vi "GetObjectStatus.vi"(0 "reference in":refnum<class "G#RemoteProxy.lvclass">, 2 "simple info (F)":bool, 5 "error in (no error)":errorcluster) -> (8 "full class name":string, 9 "# of users?":i32, 10 "all object names":string[](array[string]), 11 "last user":bool, 12 "# of objects":i32, 13 "class name":string, 14 "reference out":refnum<class "G#RemoteProxy.lvclass">, 15 "not a refnum?":bool, 16 "object name":string, 17 "all refs out":refnum<class "G#Object.lvclass">[](array[class]), 18 "counter?":bool, 19 "error out":errorcluster)   [LabVIEW 2017, in "G#RemoteProxy.lvclass"]
doc: "Returns information about the specified object. If simple info = true, only object info is return and not the arrays of objects.\n\nIf input reference is invalid, only information about the class is returned."
uses:
  G#RemoteProxy.lvclass
  G#Object/G#Object.lvclass
  G#RemoteProxy.lvclass/G#RemoteProxy.ctl
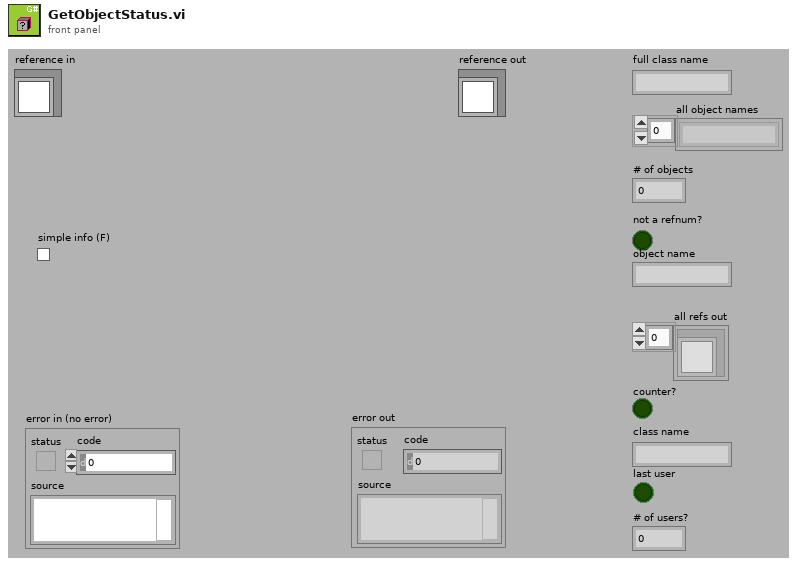
[diagram p1: front panel]
types:
  T1 = typedef "G#RemoteProxy.lvclass/ObjectAttributesRef.ctl" = refnum<data-value>
  T2 = typedef "G#RemoteProxy.lvclass/ObjectAttributesProxy.ctl" = cluster{"class hierarchy":T3[], "class name":string, "lvlib hierarchy":string[], "full class name":string, "id":u32, "owner":string, "RemoteRef":refnum<class "G#Object.lvclass">, "object name":string, "attributes":variant[], "connection ID":refnum<k5>, "address":u32, "occurrence":refnum<k4>, "ProxyClassRef":refnum<class "G#RemoteProxy.lvclass">, "InMemory?":bool, "ToString":string}
  T3 = typedef "G#Object.lvclass/G#Object_ClassHierarchy.ctl" = cluster{"ClassName":string, "FullClassName":string, "ClassPath":path, "IsLeaf":bool}
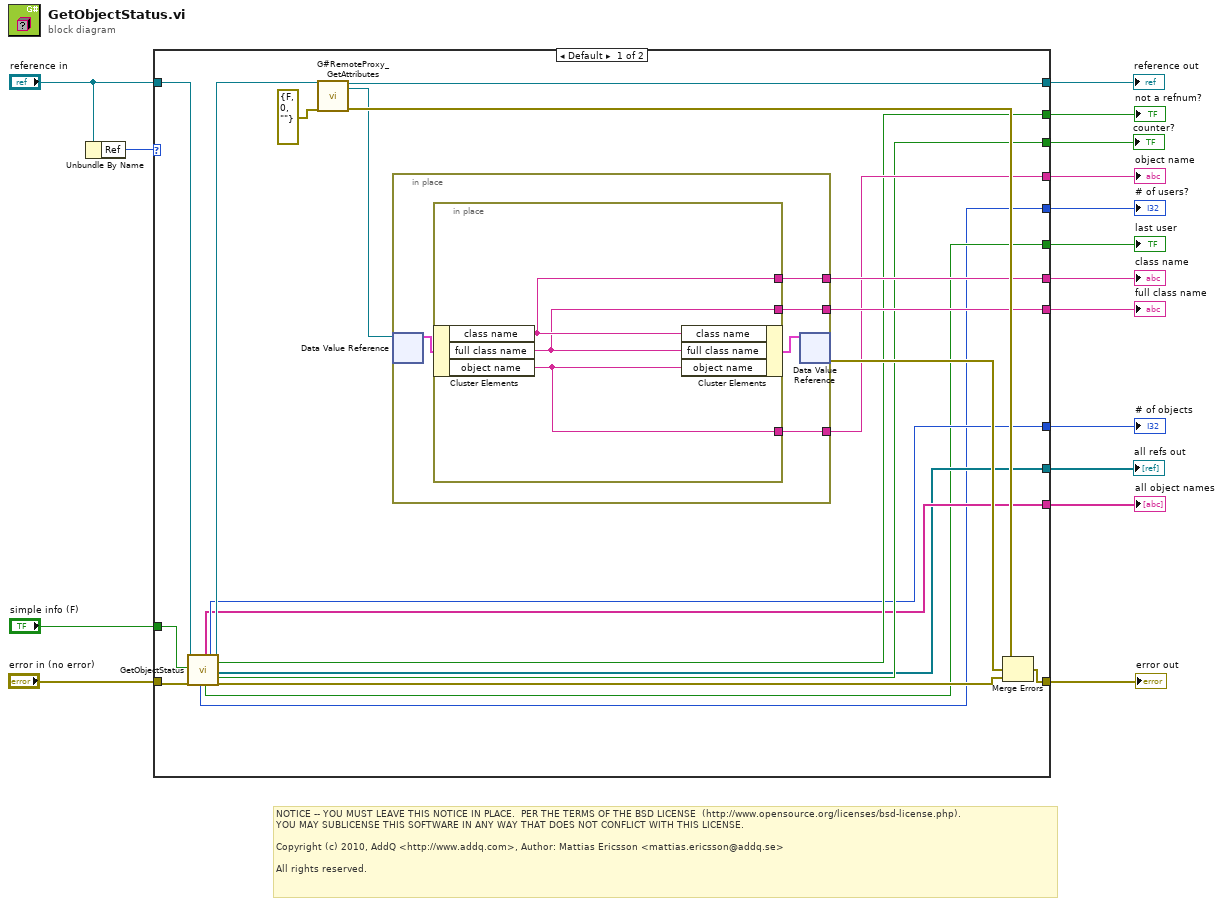
[diagram p0: block diagram]
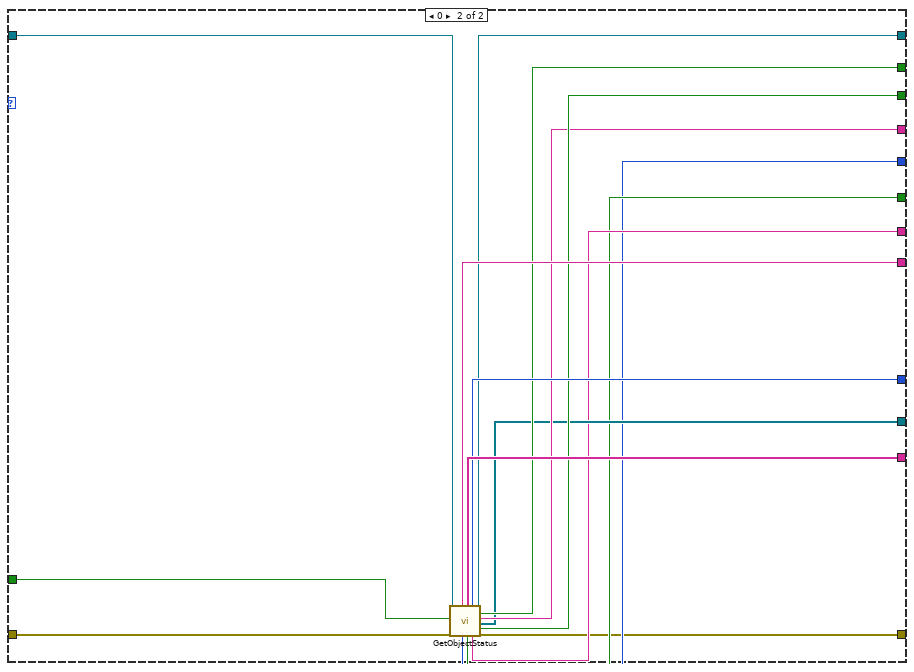
[diagram p2: hidden frame]
diagram:
  # "NOTICE -- YOU MUST LEAVE THIS NOTICE IN PLACE.  PER THE TERMS OF THE BSD LICENSE  (http://www.opensource.org/licenses/bsd-license.php).\nYOU MAY SUBLICENSE THIS SOFTWARE IN ANY WAY THAT DOES NOT CONFLICT WITH THIS LICENSE.\n\nCopyright (c) 2010, AddQ <http://www.addq.com>, Author: Mattias Ericsson <mattias.ericsson@addq.se>\n\nAll rights reserved."
  n1 = Unbundle By Name("reference in") -> ("Ref"=w15:u32)
  n2 = case shown="Default" w15 {
    tunnel: "reference in" -> [w27 w59]
    tunnel: "error in (no error)" -> [w28 w60]
    tunnel: "simple info (F)" -> [w20 w58]
    tunnel: [w30 w57] -> w12
    tunnel: [w21 w56] -> w11
    tunnel: [w22 w55] -> w10
    tunnel: [w37 w54] -> w9
    tunnel: [w24 w53] -> w8
    tunnel: [w23 w52] -> w7
    tunnel: [w29 w51] -> w6
    tunnel: [w19 w50] -> w5
    tunnel: [w31 w49] -> w4
    tunnel: [w18 w48] -> w3
    tunnel: [w17 w47] -> w2
    tunnel: [w36 w46] -> w1
    frame Default {
      n3 = call-parent "GetObjectStatus.vi"("reference in"=w27, "simple info (F)"=w20, "error in (no error)"=w28) -> ("# of users?"=w17:i32, "all object names"=w21:string[], "last user"=w18:bool, "# of objects"=w22:i32, "reference out"=w26:refnum<class "G#RemoteProxy.lvclass">, "not a refnum?"=w24:bool, "all refs out"=w19:refnum<class "G#Object.lvclass">[], "counter?"=w23:bool, "error out"=w25:errorcluster)  [unwired: 5 in, 3 out]
      n4 = call "G#RemoteProxy_GetAttributes.vi"("reference in"=w26, "error in (no error)"=errorcluster {"status"=FALSE, "code"=0, "source"=""}) -> ("reference out"=w37:refnum<class "G#RemoteProxy.lvclass">, "attributes ref"=w32:T1, "error out"=w33:errorcluster)  [unwired: 14 in, 1 out]
      n5 = in-place {
        in-place-border: [w40] -> w31
        in-place-border: [w39] -> w30
        in-place-border: [w38] -> w29
        n6 = in-place-dvr #1(w32) -> (w41:T2)  [unwired: 1 out]
        n7 = in-place {
          in-place-border: [w45] -> w40
          in-place-border: [w44] -> w39
          in-place-border: [w43] -> w38
          n8 = in-place-cluster #2(w41) -> ("class name"=w45:string, "full class name"=w44:string, "object name"=w43:string)
          n9 = in-place-cluster #2("class name"=w45, "full class name"=w44, "object name"=w43) -> (w42:T2)
        }
        n10 = in-place-dvr #1(w42) -> (w34:errorcluster)  [unwired: 1 out]
      }
      n11 = Merge Errors(w33, w34, w25) -> (w36:errorcluster)
    }
    frame 0 {
      n12 = call-parent "GetObjectStatus.vi"("reference in"=w59, "simple info (F)"=w58, "error in (no error)"=w60) -> ("full class name"=w57:string, "# of users?"=w47:i32, "all object names"=w56:string[], "last user"=w48:bool, "# of objects"=w55:i32, "class name"=w49:string, "reference out"=w54:refnum<class "G#RemoteProxy.lvclass">, "not a refnum?"=w53:bool, "object name"=w51:string, "all refs out"=w50:refnum<class "G#Object.lvclass">[], "counter?"=w52:bool, "error out"=w46:errorcluster)  [unwired: 5 in]
    }
  }
  "reference out" <- w9
  "# of users?" <- w2
  "last user" <- w3
  "all refs out" <- w5
  "not a refnum?" <- w8
  "# of objects" <- w10
  "class name" <- w4
  "object name" <- w6
  "all object names" <- w11
  "counter?" <- w7
  "full class name" <- w12
  "error out" <- w1
